vi "state control.vi"(9 "Datalog directory path":path, 10 "Plant Mode of Operation":T1=enum."Automatic Operation", 11 "Operator Selected State":u16(ring)=1) -> (0 "Range error":bool, 1 "Elapsed time in current state":dbl format="%.2f", 3 "Plant State out":u16(ring)=1)   [LabVIEW 2019]
uses:
  Plant mode.ctl
  DAQ configuration/Sensor buffer command.ctl
  logic buffer cmd.ctl
panel:
  in  "Tab Control":enum32{"Inputs", "Outputs"}(tab)
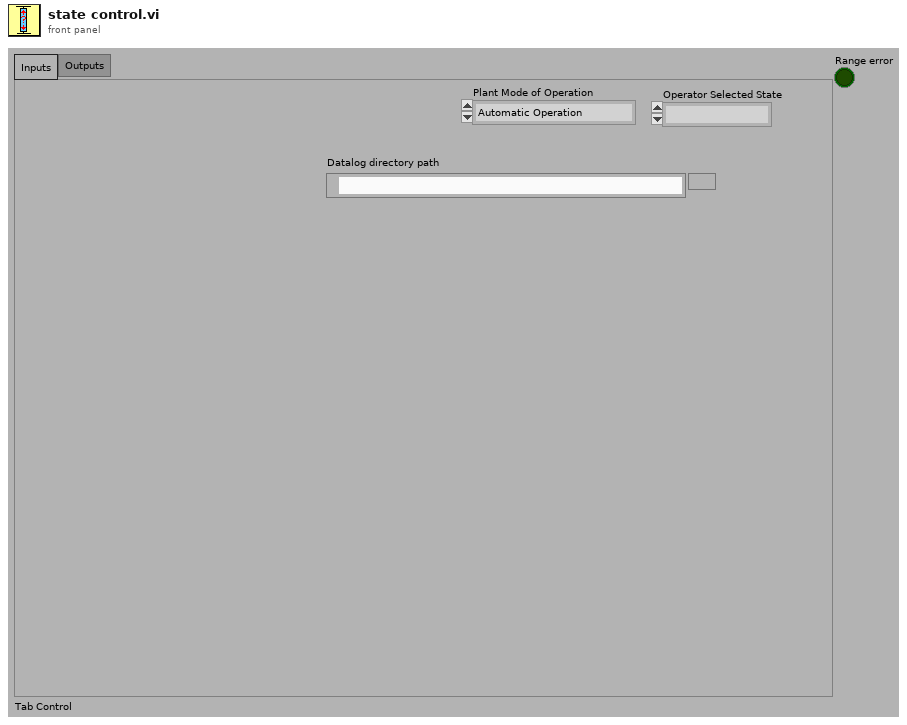
[diagram p1: front panel]
types:
  T1 = typedef "Plant mode.ctl" = enum16{"Manual Locked in State", "Automatic Operation"}
  T2 = typedef "logic buffer cmd.ctl" = enum16{"read", "write ouput settings", "write rules", "write setpoints", "write output descriptions", "write all", "calculate setpoints", "save", "open", "Load all setpoint code", "Load one setpoint code", "Configure one setpoint code"}
  T3 = typedef "Sensor buffer command.ctl" = enum16{"read average", "read recent", "read all", "write", "set buffer size", "Read channel config", "Write channel config", "clear"}
  T4 = typedef "Sensor data.ctl" = cluster{" Sensor array":T5[], "Time":dbl}
  T5 = typedef "sensor cluster.ctl" = cluster{"voltage":sgl, "scaled":sgl, "units":string, "Out of Range":bool}
  T6 = typedef "Plant state.ctl" = u16
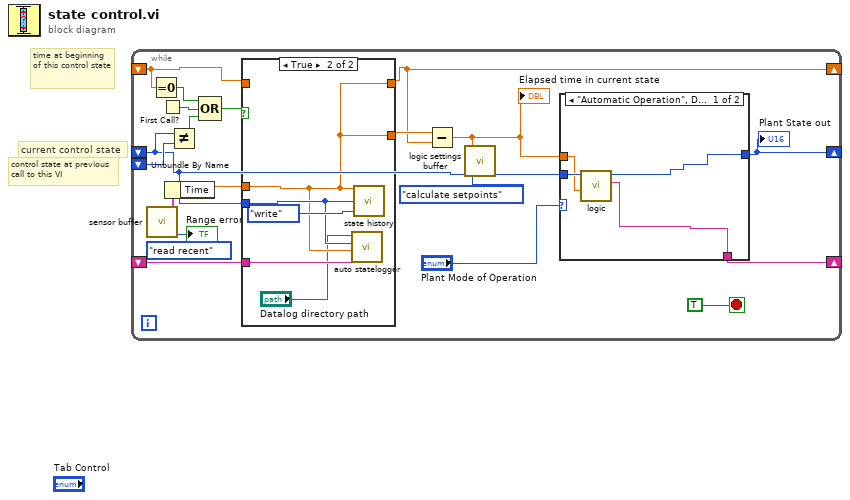
[diagram p0: block diagram]
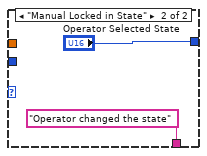
[diagram p3: hidden frame]
diagram:
  # "current control state"
  # "control state at previous call to this VI"
  # "time at beginning of this control state"
  n1 = while {
    shift-left: _ -> [w12]
    shift-right: [w13] -> _
    shift-left: _ -> [w18]
    shift-left: _ -> [w3]
    shift-right: [w6] -> _
    shift-right: [w7] -> _
    shift-left: _ -> [w16]
    stop <- TRUE stop-if-true
    n2 = call "sensor buffer.vi"("command"=Sensor_buffer_command."read recent") -> ("Range error"=→"Range error":bool, "Calibrated data"=w19:T4)  [unwired: 6 in, 3 out]
    n3 = Equal To 0?(x=w12) -> (x = 0?=w11:bool)
    n4 = First Call?() -> (First Call?: T/F=w10:bool)
    n5 = Unbundle By Name(w19) -> ("Time"=w15:dbl)
    n6 = Not Equal?(x=w3, y=w18) -> (x != y?=w9:bool)
    n7 = Compound Arithmetic op=OR(w11, w10, w9) -> (w8:bool)
    n8 = case shown="True" w8 {
      tunnel: w15 -> [w23 w25]
      tunnel: w3 -> [_ w27]
      tunnel: w16 -> [_ w26]
      tunnel: [w23 w25] -> w14
      tunnel: [w22 w25] -> w13
      tunnel: w12 -> [w22 _]
      frame False {
      }
      frame True {
        n9 = call "auto statelogger.vi"("Rule name"=w26, "Time"=w25, "Plant State"=w27, "Datalog directory path"="Datalog directory path") -> ()  [unwired: 7 in, 1 out]
        n10 = call "state history.vi"("command"=enum16{"write", "read", "reset"}."write", "Plant State"=w27, "Time"=w25) -> ()  [unwired: 1 out]
      }
    }
    n11 = Subtract(x=w14, y=w13) -> (x-y=w4:dbl)
    "Elapsed time in current state" <- w4
    n12 = call "logic settings buffer.vi"("Plant  state"=w3, "Elapsed time in current state"=w4, "command"=logic_buffer_cmd."calculate setpoints") -> ("Plant  state out"=w2:u16)  [unwired: 9 in, 7 out]
    n13 = case shown="\"Automatic Operation\", Default" "Plant Mode of Operation" {
      tunnel: [w30 "Operator Selected State"] -> w6
      tunnel: w2 -> [w32 _]
      tunnel: w4 -> [w31 _]
      tunnel: [w29 "Operator changed the state" ("Rule name")] -> w7
      frame "Automatic Operation", Default {
        n14 = call "logic.vi"("Elapsed time in current state"=w31, "Plant State in"=w32) -> ("Rule name"=w29:string, "Plant State out"=w30:T6)  [unwired: 8 in]
      }
      frame "Manual Locked in State" {
      }
    }
    "Plant State out" <- w6
  }
